vi "WriteData.vi"(4 "Station":T1(ring), 6 "TableName":string, 8 "error in (no error)":errorcluster, 9 "column information":T2[](array[typedef]), 10 "data":variant, 11 "DataBase in":refnum<class "DataBase.lvclass">) -> (0 "error out":errorcluster, 3 "DataBase out":refnum<class "DataBase.lvclass">)   [LabVIEW 2019, in "DataBase.lvlib" / "DataBase.lvclass"]
uses:
  DataBase.lvclass
  <vilib>/addons/database/Auxilliary.llb/DB Tools Column Info.ctl
  <vilib>/addons/database/Auxilliary.llb/DB Tools DataTypes.ctl
  DataBase.lvclass/DataBase.ctl
  <vilib>/addons/database/NI_Database_API.lvlib
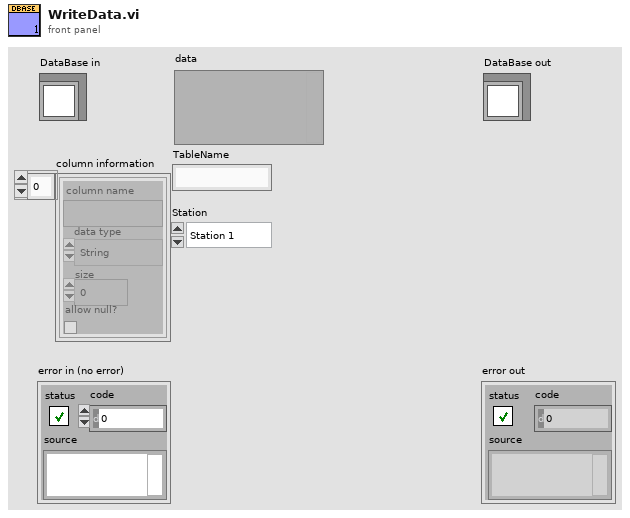
[diagram p1: front panel]
types:
  T1 = enum16{"Station 1", "Station 2", "Station 3", "Station 4"}
  T2 = typedef "NI_Database_API.lvlib/DB Tools Column Info.ctl" = cluster{"column name":string, "data type":T3, "size":i32, "allow null?":bool}
  T3 = typedef "NI_Database_API.lvlib/DB Tools DataTypes.ctl" = enum16{"String", "Long (I32)", "Single (SGL)", "Double (DBL)", "Date/Time", "Binary"}
  T4 = typedef "NI_Database_API.lvlib/Conn ObjectReference.ctl" = refnum<k1>
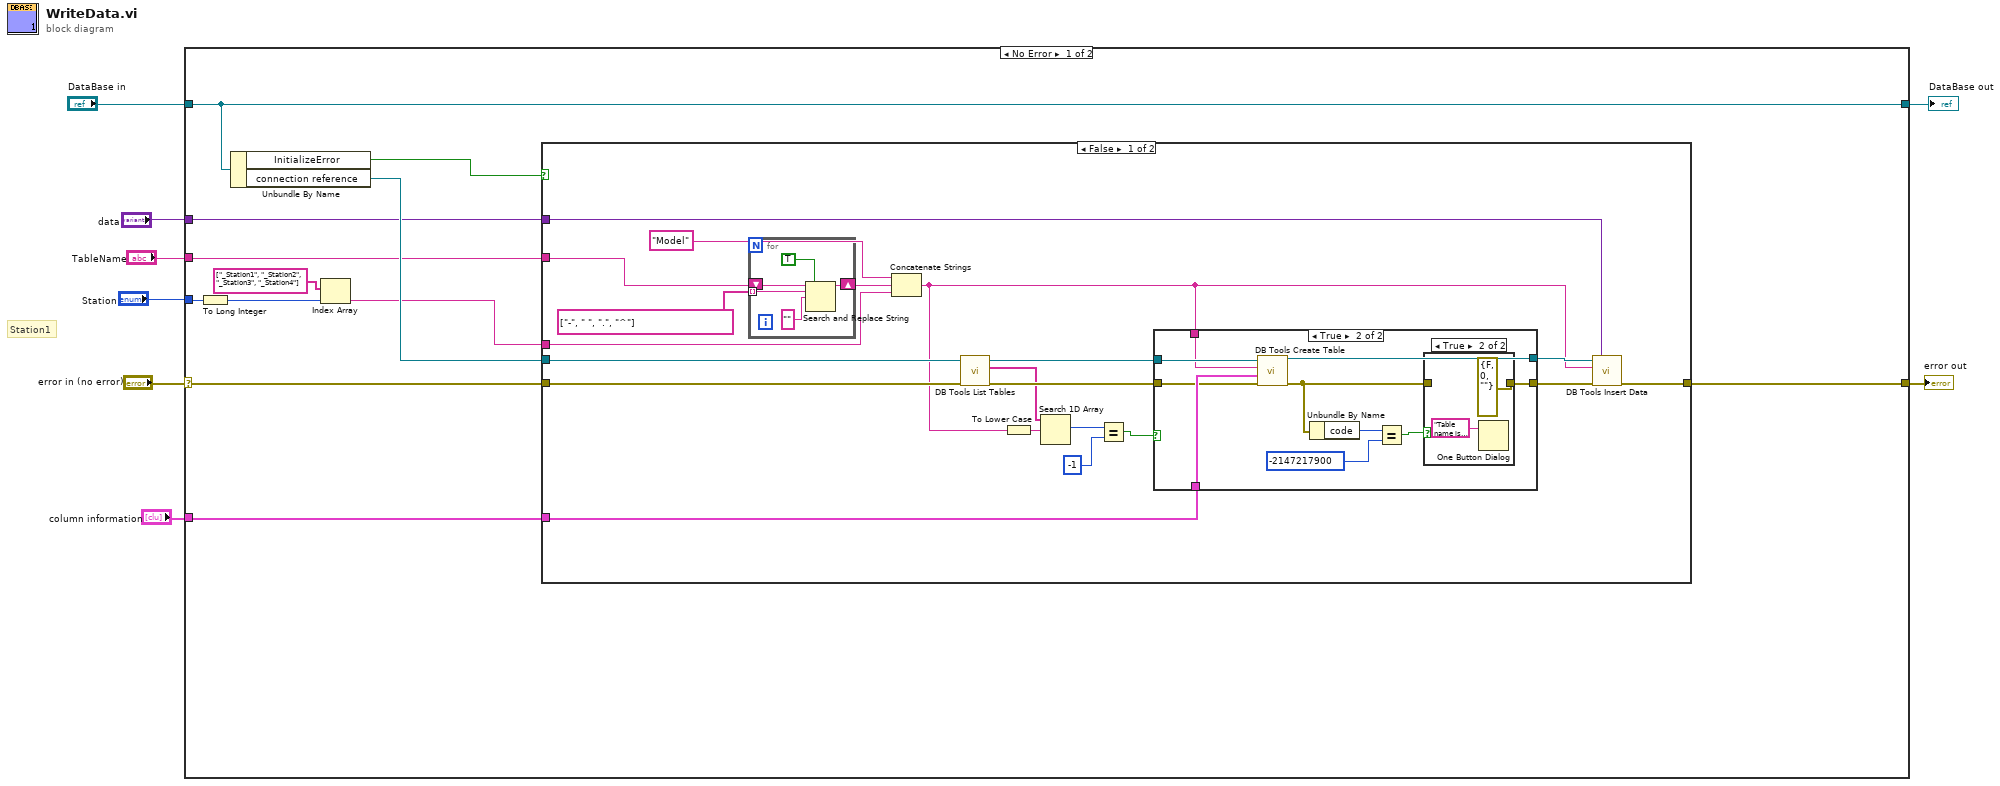
[diagram p0: block diagram]
diagram:
  # "Station1"
  n1 = case shown="No Error" "error in (no error)" {
    selector: "error in (no error)" -> [w16 w63]
    tunnel: [w15 w63] -> w7
    tunnel: [w20 w62] -> w5
    tunnel: "DataBase in" -> [w20 w62]
    tunnel: "column information" -> [w18 _]
    tunnel: "data" -> [w17 _]
    tunnel: "TableName" -> [w14 _]
    tunnel: "Station" -> [w12 _]
    frame No Error {
      n2 = To Long Integer(number=w12) -> (32bit integer=w11:i32)
      n3 = Unbundle By Name(w20) -> ("InitializeError"=w13:bool, "connection reference"=w19:T4)
      n4 = Index Array(array=string[] ["_Station1", "_Station2", "_Station3", "_Station4"], index=w11) -> (element=w9:string)
      n5 = case shown="False" w13 {
        tunnel: w19 -> [w31 _]
        tunnel: w18 -> [w30 _]
        tunnel: w17 -> [w29 _]
        tunnel: w16 -> [w28 w61]
        tunnel: [w27 w61] -> w15
        tunnel: w14 -> [w26 _]
        tunnel: w9 -> [w21 _]
        frame False {
          n6 = for {
            tunnel: string[] ["-", " ", ".", "^"] -> [w45] mode=indexing
            shift-right: [w42] -> w24
            shift-left: w26 -> [w43]
            n7 = Search and Replace String(replace all?=TRUE ("replace all? (F)"), input string=w43, search string=w45, replace string="" ("replace string (\"\")")) -> (result string=w42:string)  [unwired: 4 in, 3 out]
          }
          n8 = Concatenate Strings("Model" ("string"), w24, w21) -> (w23:string)
          n9 = call <vilib>:"DB Tools List Tables.vi"("error in (no error)"=w28, "connection reference"=w31) -> ("error out"=w37:errorcluster, "tables"=w36:string[], "connection reference out"=w38:T4)  [unwired: 3 in]
          n10 = To Lower Case(string=w23) -> (all lower case string=w32:string)
          n11 = Search 1D Array(1D array=w36, element=w32) -> (index of element=w35:i32)  [unwired: 1 in]
          n12 = Equal?(x=w35, y=-1) -> (x = y?=w33:bool)
          n13 = case shown="True" w33 {
            tunnel: [w46 w48] -> w40
            tunnel: [w47 w57] -> w39
            tunnel: w30 -> [_ w56]
            tunnel: w38 -> [w47 w55]
            tunnel: w37 -> [w46 w54]
            tunnel: w23 -> [_ w53]
            frame False {
            }
            frame True {
              n14 = call <vilib>:"DB Tools Create Table.vi"("error in (no error)"=w54, "column information"=w56, "table"=w53, "connection reference"=w55) -> ("error out"=w49:errorcluster, "connection reference out"=w57:T4)  [unwired: 4 in]
              n15 = Unbundle By Name(w49) -> ("code"=w52:i32)
              n16 = Equal?(x=w52, y=-2147217900) -> (x = y?=w50:bool)
              n17 = case shown="True" w50 {
                tunnel: w49 -> [w58 _]
                tunnel: [w58 errorcluster {"status"=FALSE, "code"=0, "source"=""} ("error out")] -> w48
                frame False {
                }
                frame True {
                  n18 = One Button Dialog(message="Table name is not allow!") -> ()  [unwired: 1 in, 1 out]
                }
              }
            }
          }
          n19 = call <vilib>:"DB Tools Insert Data.vi"("data"=w29, "error in (no error)"=w40, "table"=w23, "connection reference"=w39) -> ("error out"=w27:errorcluster)  [unwired: 6 in, 1 out]
        }
        frame True {
        }
      }
    }
    frame Error {
    }
  }
  "error out" <- w7
  "DataBase out" <- w5
